vi "checkListOfRegMsg.vi"(8 "error in (no error)":errorcluster, 9 "msgName":string="M1M3", 10 "compName":string="M1M3", 11 "tcpServerBase in":refnum<class "TcpServerBase.lvclass">) -> (0 "error out":errorcluster, 2 "msgRegistered?":bool, 3 "tcpServerBase out":refnum<class "TcpServerBase.lvclass">)   [LabVIEW 2018, in "TcpServerBase.lvclass"]
doc: "Check if incoming message (event/telemetry) is registered."
uses:
  TcpServerBase.lvclass
  TcpServerBase.lvclass/TcpServerBase.ctl
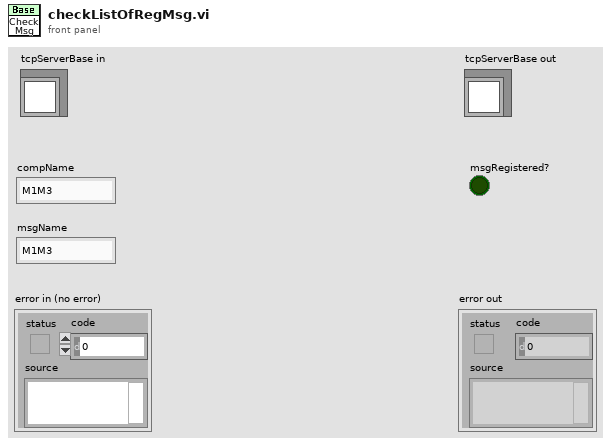
[diagram p1: front panel]
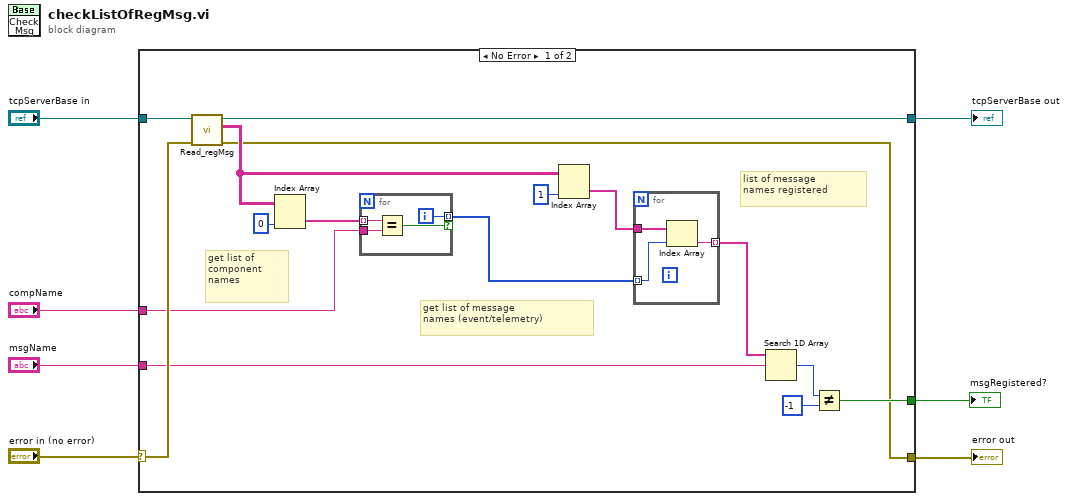
[diagram p0: block diagram]
diagram:
  n1 = case shown="No Error" "error in (no error)" {
    selector: "error in (no error)" -> [w17 w32]
    tunnel: [w8 w32] -> w6
    tunnel: [w19 w31] -> w4
    tunnel: "tcpServerBase in" -> [w20 w31]
    tunnel: [w21 _] -> w3
    tunnel: "compName" -> [w15 _]
    tunnel: "msgName" -> [w9 _]
    frame No Error {
      # "list of message \nnames registered"
      # "get list of message\nnames (event/telemetry)"
      # "get list of \ncomponent\nnames"
      n2 = call "Read_regMsg.vi"("error in (no error)"=w17, "TcpServerBase in"=w20) -> ("error out"=w8:errorcluster, "regMsg"=w13:string[][], "TcpServerBase out"=w19:refnum<class "TcpServerBase.lvclass">)  [unwired: 7 in]
      n3 = Index Array(array=w13, index (col)=0 ("index (row)")) -> (element=w16:string[])  [unwired: 1 in]
      n4 = for {
        tunnel: w15 -> [w30]
        tunnel: w16 -> [w29] mode=indexing
        tunnel: [w28] -> w11 mode=indexing if=w27
        i -> [w28]
        n5 = Equal?(x=w29, y=w30) -> (x = y?=w27:bool)
      }
      n6 = Index Array(array=w13, index (col)=1 ("index (row)")) -> (element=w12:string[])  [unwired: 1 in]
      n7 = for {
        tunnel: w12 -> [w26]
        tunnel: w11 -> [w24] mode=indexing
        tunnel: [w25] -> w10 mode=indexing
        n8 = Index Array(array=w26, index=w24) -> (element=w25:string)
      }
      n9 = Search 1D Array(1D array=w10, element=w9) -> (index of element=w23:i32)  [unwired: 1 in]
      n10 = Not Equal?(x=w23, y=-1) -> (x != y?=w21:bool)
    }
    frame Error {
    }
  }
  "error out" <- w6
  "tcpServerBase out" <- w4
  "msgRegistered?" <- w3
